vi "Creators Status Created Events.vi"(11 "Template Event in":refnum<class "Template Event.lvclass">) -> (0 "Created Event Count":i32, 1 "Created Event Aliases":string[](array[string]), 2 "Created Event Exist?":bool, 3 "Template Event out":refnum<class "Template Event.lvclass">)   [LabVIEW 2021, in "_Template.lvlib" / "Templates.lvlib" / "Template Event.lvlib" / "Template Event.lvclass"]
uses:
  Template Event.lvclass
  Template Event.lvclass/Template Event.ctl
  <vilib>/jettl/jettl/jettl/Event/Event.lvclass
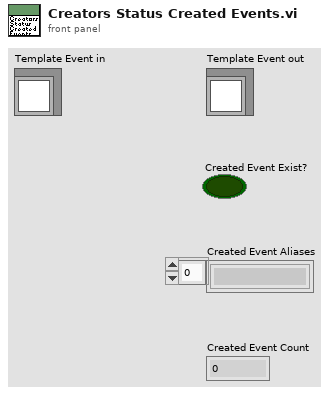
[diagram p1: front panel]
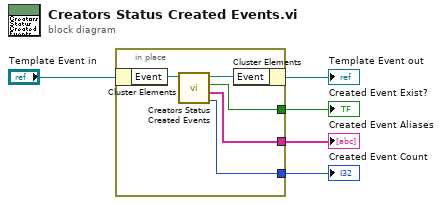
[diagram p0: block diagram]
diagram:
  n1 = in-place {
    in-place-border: [w8] -> w3
    in-place-border: [w7] -> w2
    in-place-border: [w6] -> w1
    n2 = in-place-cluster #1("Template Event in") -> ("Event"=w10:refnum<class "Event.lvclass">)
    n3 = call-dynamic "Creators Status Created Events.vi"("Event in"=w10) -> ("Created Event Count"=w7:i32, "Created Event Aliases"=w6:string[], "Created Event Exist?"=w8:bool, "Event out"=w9:refnum<class "Event.lvclass">)  [unwired: 7 in]
    n4 = in-place-cluster #1("Event"=w9) -> (→"Template Event out":refnum<class "Template Event.lvclass">)
  }
  "Created Event Aliases" <- w1
  "Created Event Count" <- w2
  "Created Event Exist?" <- w3
